vi "常规五参数关键参数区.vi"(11 "数组":u16[](array[numeric]) format="%04xH") -> (3 "关键参数区":T1)   [LabVIEW 2016, in "斯坦道多参数.lvlib"]
panel:
  # "共占用19字"
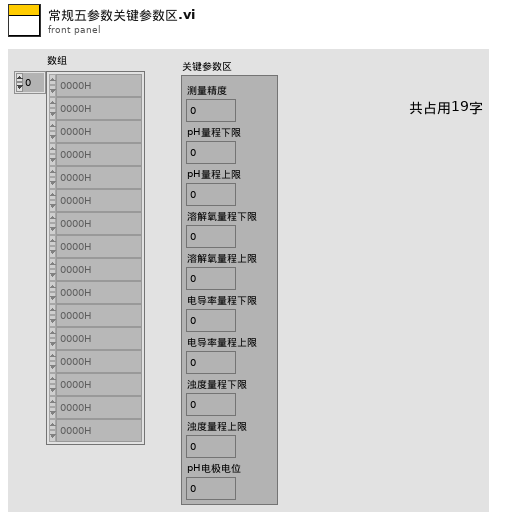
[diagram p1: front panel]
types:
  T1 = cluster{"测量精度":u16, "pH量程下限":sgl, "pH量程上限":sgl, "溶解氧量程下限":sgl, "溶解氧量程上限":sgl, "电导率量程下限":sgl, "电导率量程上限":sgl, "浊度量程下限":sgl, "浊度量程上限":sgl, "pH电极电位":sgl}
  T2 = cluster{"WORD":u16, "FLOAT":sgl, "FLOAT":sgl, "FLOAT":sgl, "FLOAT":sgl, "FLOAT":sgl, "FLOAT":sgl, "FLOAT":sgl, "FLOAT":sgl, "FLOAT":sgl}
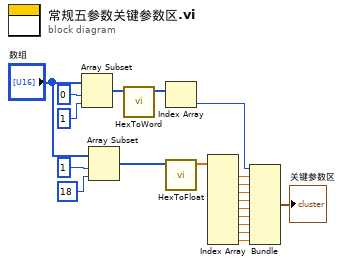
[diagram p0: block diagram]
diagram:
  n1 = Array Subset(array="数组", index=0 ("索引"), length=1 ("长度")) -> (w17:u16[])
  n2 = Array Subset(array="数组", index=1 ("索引"), length=18 ("长度")) -> (w13:u16[])
  n3 = call "HexToWord.vi"("数组"=w17) -> ("WORD"=w16:u16[])  [unwired: 10 in]
  n4 = Index Array(array=w16) -> (element=w18:u16)  [unwired: 1 in]
  n5 = call "HexToFloat.vi"("数组"=w13) -> ("FLOAT"=w12:sgl[])  [unwired: 10 in]
  n6 = Index Array(array=w12) -> (element #1=w11:sgl, element #2=w10:sgl, element #3=w9:sgl, element #4=w8:sgl, element #5=w6:sgl, element #6=w5:sgl, element #7=w4:sgl, element #8=w3:sgl, element #9=w2:sgl)  [unwired: 9 in]
  n7 = Bundle("WORD"=w18, "FLOAT"=w11, "FLOAT"=w10, "FLOAT"=w9, "FLOAT"=w8, "FLOAT"=w6, "FLOAT"=w5, "FLOAT"=w4, "FLOAT"=w3, "FLOAT"=w2) -> (→"关键参数区":T2)  [unwired: 1 in]
